vi "Add Turn Stats.vi"(8 "error in (no error)":errorcluster, 10 "Team Stats":T1, 11 "Team in":refnum<class "Team.lvclass">) -> (0 "error out":errorcluster, 3 "Team out":refnum<class "Team.lvclass">)   [LabVIEW 2020, in "SquareBattle.lvlib" / "Team.lvclass"]
uses:
  Team.lvclass
  Team Stats.ctl
  Team.lvclass/Team.ctl
  SquareBattle.lvlib
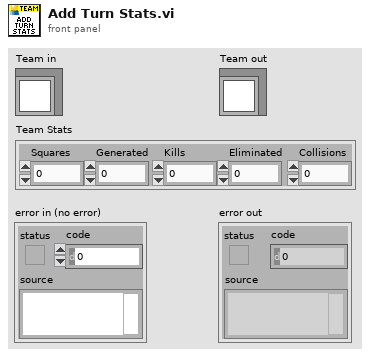
[diagram p1: front panel]
types:
  T1 = typedef "SquareBattle.lvlib/Team Stats.ctl" = cluster{"Squares":i32, "Generated":i32, "Kills":i32, "Eliminated":i32, "Collisions":i32}
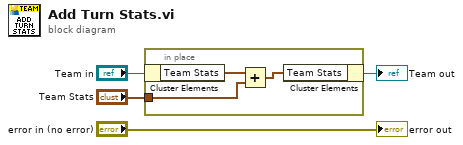
[diagram p0: block diagram]
diagram:
  n1 = in-place {
    in-place-border: "Team Stats" -> [w6]
    n2 = in-place-cluster #1("Team in") -> ("Team Stats"=w7:T1)
    n3 = Add(x=w7, y=w6) -> (x+y=w5:T1)
    n4 = in-place-cluster #1("Team Stats"=w5) -> (→"Team out":refnum<class "Team.lvclass">)
  }
  "error out" <- "error in (no error)"
